vi "SeCrTs-RD globals.vi"() -> ()   [LabVIEW 2022 SP3]
panel:
  in  "Ip":string
  in  "Log time":dbl
  out "C/NC":bool
  in  "reader":refnum<k21>
  out "Connect?":bool
  in  "writer url":refnum<k21>
  out "EXIT":bool
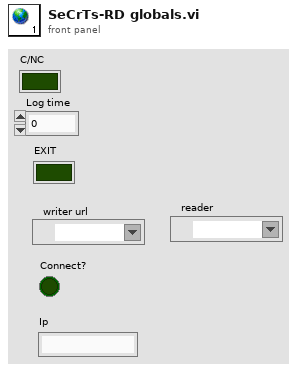
[diagram p1: front panel]
diagram:
